vi "Update Status.vi"(9 "Spec Page Interface":T1, 11 "TwoTasksMetaDataObj in":refnum<class "FixedChannelTBModuleDecideFeatures.lvclass">) -> ()   [LabVIEW 2013, in "FixedChannelTBModuleDecideFeatures.lvclass"]
uses:
  FixedChannelTBModuleDecideFeatures.lvclass
  <resource>/dialog/NewProjectWizard/Spec Page Interface.ctl
  <resource>/dialog/NewProjectWizard/MetaDataObj/MetaDataObj.lvclass/MetaDataObj.ctl
  FixedChannelTBModuleDecideFeatures.lvclass/FixedChannelTBModuleDecideFeatures.ctl
  <resource>/dialog/NewProjectWizard/MetaDataObj/Accessors/Read Project Name.vi
  <resource>/dialog/NewProjectWizard/MetaDataObj/Accessors/Read Project Root.vi
  <resource>/dialog/NewProjectWizard/MetaDataObj/Accessors/Read File Prefix.vi
  Read Channel Specification.vi
panel:
  in  "Please choose a different name.":string="Please choose a different name."
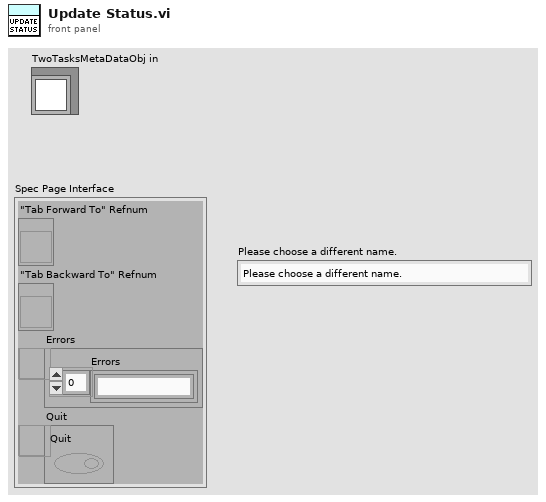
[diagram p1: front panel]
types:
  T1 = typedef "Spec Page Interface.ctl" = cluster{"\"Tab Forward To\" Refnum":refnum<vi>, "\"Tab Backward To\" Refnum":refnum<vi>, "Errors":refnum<user-event>, "Quit":refnum<user-event>}
  T2 = typedef "FixedChannelTBModuleDecideFeatures.lvclass/channel configuration.ctl" = cluster{"Name":string, "channel classification":T3, "data type":T4}
  T3 = typedef "TBM channel.lvclass/channel classification.ctl" = enum16{"input data", "output data", "processing parameter", "processing result"}
  T4 = typedef "tag bus.lvlib/tag descriptor.lvclass/Data Type.ctl" = enum16{"Double", "Single", "I64", "I32", "I16", "I8", "U64", "U32", "U16", "U8", "Boolean", "String", "Array of Double", "Array of Single", "Array of I64", "Array of I32", "Array of I16", "Array of I8", "Array of U64", "Array of U32", "Array of U16", "Array of U8", "Array of Boolean", "Array of String"}
  T5 = enum8{"Enabled", "Disabled", "Disabled and Grayed Out"}
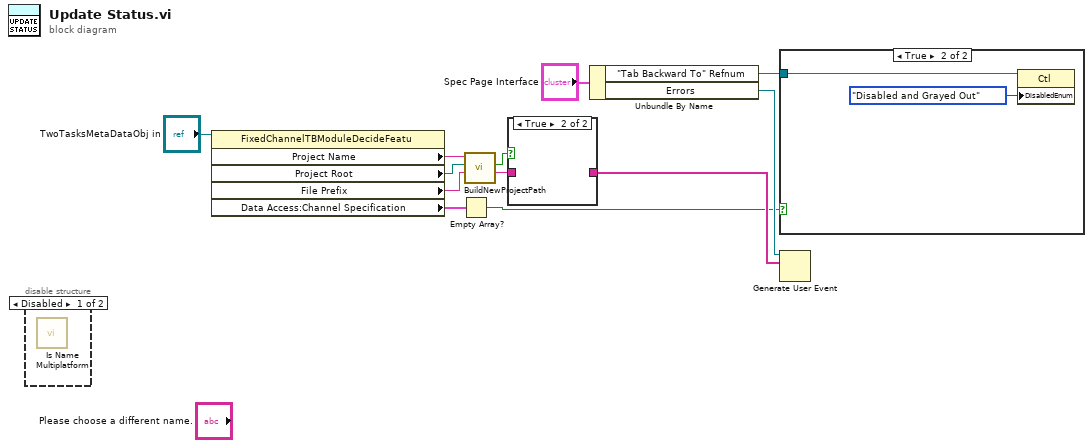
[diagram p0: block diagram]
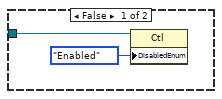
[diagram p2: hidden frame]
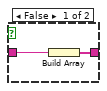
[diagram p4: hidden frame]
diagram:
  n1 = disable-structure shown="Disabled" {
    frame Disabled {
      n2 = call <vilib>:"Is Name Multiplatform.vi"() -> ()  [unwired: 7 in, 5 out]
    }
    frame Enabled {
    }
  }
  n3 = property class="FixedChannelTBModuleDecideFeatu"(reference="TwoTasksMetaDataObj in") -> ("Project Name"=w8:string, "Project Root"=w9:path, "File Prefix"=w7:string, "Data Access:Channel Specification"=w3:T2[])  [unwired: 1 in, 2 out]
  n4 = Empty Array?(array=w3) -> (empty?=w1:bool)
  n5 = call <resource>:"BuildNewProjectPath.vi"("File Prefix"=w7, "Project Root"=w9, "Project Name"=w8) -> ("Error Message"=w5:string, "Valid?"=w6:bool)  [unwired: 6 in, 1 out]
  n6 = case shown="True" w6 {
    tunnel: w5 -> [w14 _]
    tunnel: [w13 _] -> w4
    frame False {
      n7 = Build Array(w14) -> (w13:string[])
    }
    frame True {
    }
  }
  n8 = Unbundle By Name("Spec Page Interface") -> ("\"Tab Backward To\" Refnum"=w2:refnum<vi>, "Errors"=w11:refnum<user-event>)
  n9 = case shown="True" w1 {
    tunnel: w2 -> [w16 w18]
    frame False {
      n10 = property class="Ctl"(reference=w16, "DisabledEnum"=T5."Enabled" ("Disabled")) -> ()  [unwired: 1 in, 2 out]
    }
    frame True {
      n11 = property class="Ctl"(reference=w18, "DisabledEnum"=T5."Disabled and Grayed Out" ("Disabled")) -> ()  [unwired: 1 in, 2 out]
    }
  }
  n12 = Generate User Event(user event=w11, event data cluster=w4) -> ()  [unwired: 2 in, 2 out]
